vi "LeCroy Test Driver V2.vi"() -> ()   [LabVIEW 2013]
doc: "This example shows how to configure the oscilloscope to perform an edge-triggered waveform acquisition."
uses:
  Sub VI's/Settings_TypeDef.ctl
  <instrlib>/LeCroy Wave Series/LeCroy Wave Series.lvlib
panel:
  in  "Settings":T1={"LeCroy IP"="169.254.20.90", "Ch1"={"On/Off"=FALSE, "Bandwidth (Dropdown)"=0, "Vertical Range (V)"=0.2, "Vertical Offset (V)"=0.0}, "Ch2"={"On/Off"=TRUE, "Bandwidth (Dropdown)"=0, "Vertical Range (V)"=1.2, "Vertical Offset (V)"=0.0}, "Ch3"={"On/Off"=TRUE, "Bandwidth (Dropdown)"=0, "Vertical Range (V)"=0.2, "Vertical Offset (V)"=0.0}, "Ch4"={"On/Off"=FALSE, "Bandwidth (Dropdown)"=0, "Vertical Range (V)"=0.2, "Vertical Offset (V)"=0.0}, "T axis"={"Time base (s/div)"=0.0002, "Time offset (s)"=0.0, "Max Sample Points"=5000}, "Trig"={"Trigger mode"=2, "Trigger Slope"=0, "Trigger Source"=1, "Trigger Level (V)"=0.04}, "Timeout (ms)"=10000.0} {"Trig"."Trigger mode" items=["Auto", "Normal", "Single", "Single, auto trigger"]; "Trig"."Trigger Slope" items=["Rising", "Falling"]; "Trig"."Trigger Source" items=["Channel 1", "Channel 2", "Channel 3", "Channel 4", "External", "Power Line"]; "Trig"."Trigger Level (V)" format="%#_6p"; "T axis"."Max Sample Points" format="%.0p" items=["50"=50, "100"=100, "250"=250, "500"=500, "1000"=1000, "2500"=2500, "5K"=5000, "10K"=10000, "25K"=25000, "50K"=50000, "100K"=100000, "250K"=250000, "500K"=500000, "1M"=1000000, "2M"=2000000, "2.5M"=2500000, "5M"=5000000, "10M"=10000000, "25M"=25000000, "50M"=50000000, "100M"=100000000]; "T axis"."Time base (s/div)" format="%#_6p"; "Ch4"."Bandwidth (Dropdown)" items=["Full", "20MHZ", "25MHZ", "200MHZ", "250MHZ", "1GHZ", "3GHZ", "4GHZ"]; "Ch3"."Bandwidth (Dropdown)" items=["Full", "20MHZ", "25MHZ", "200MHZ", "250MHZ", "1GHZ", "3GHZ", "4GHZ"]; "Ch2"."Bandwidth (Dropdown)" items=["Full", "20MHZ", "25MHZ", "200MHZ", "250MHZ", "1GHZ", "3GHZ", "4GHZ"]; "Ch1"."Bandwidth (Dropdown)" items=["Full", "20MHZ", "25MHZ", "200MHZ", "250MHZ", "1GHZ", "3GHZ", "4GHZ"]}
  out "Configure time (ms)":u32
  out "Initilize time (ms)":u32
  out "Aquire waveform time (ms)":u32
  out "Waveform Data":waveform(dbl)[](graph)
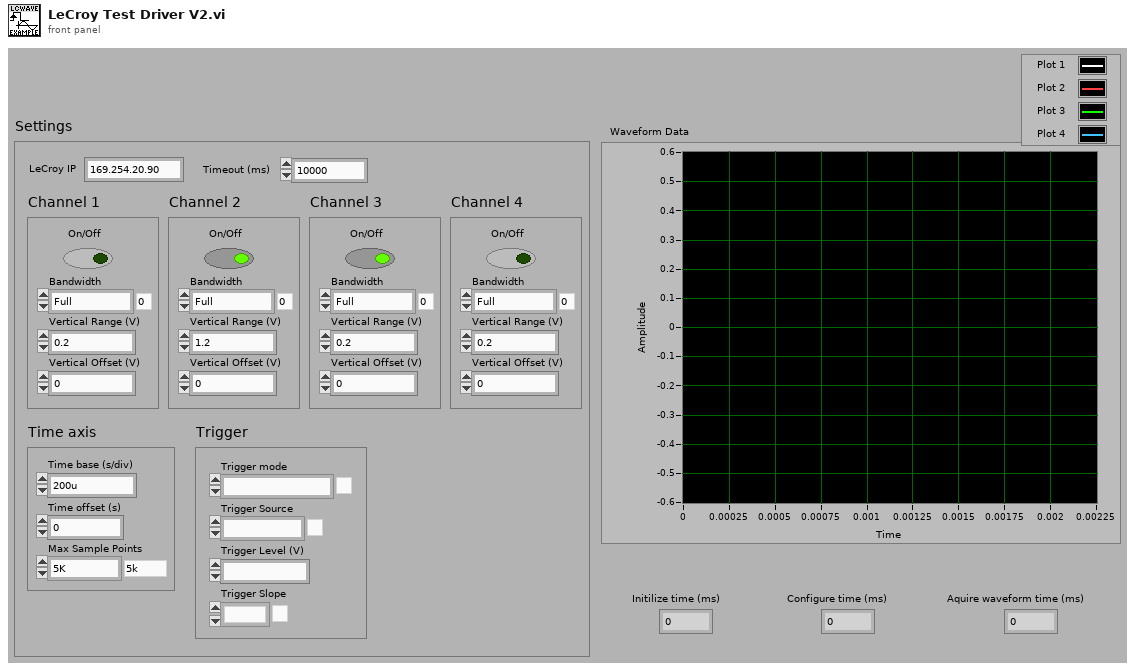
[diagram p1: front panel]
types:
  T1 = typedef "Settings_TypeDef.ctl" = cluster{"LeCroy IP":string, "Ch1":cluster{"On/Off":bool, "Bandwidth (Dropdown)":u16, "Vertical Range (V)":dbl, "Vertical Offset (V)":dbl}, "Ch2":cluster{"On/Off":bool, "Bandwidth (Dropdown)":u16, "Vertical Range (V)":dbl, "Vertical Offset (V)":dbl}, "Ch3":cluster{"On/Off":bool, "Bandwidth (Dropdown)":u16, "Vertical Range (V)":dbl, "Vertical Offset (V)":dbl}, "Ch4":cluster{"On/Off":bool, "Bandwidth (Dropdown)":u16, "Vertical Range (V)":dbl, "Vertical Offset (V)":dbl}, "T axis":cluster{"Time base (s/div)":dbl, "Time offset (s)":dbl, "Max Sample Points":i32}, "Trig":cluster{"Trigger mode":u16, "Trigger Slope":u16, "Trigger Source":u16, "Trigger Level (V)":dbl}, "Timeout (ms)":dbl}
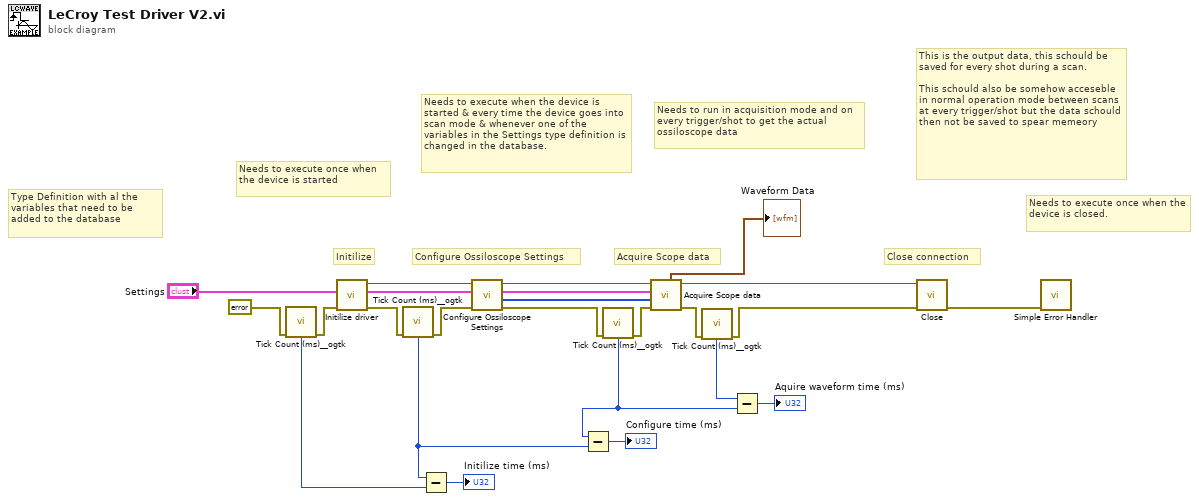
[diagram p0: block diagram]
diagram:
  # "Needs to execute once when the device is closed."
  # "This is the output data, this schould be saved for every shot during a scan.\n\nThis schould also be somehow acceseble in normal operation mode between scans at every trigger/shot but the data schould then not be saved to spear memeory"
  # "Needs to run in acquisition mode and on every trigger/shot to get the actual ossiloscope data"
  # "Needs to execute when the device is started & every time the device goes into scan mode & whenever one of the variables in the Settings type definition is changed in the database."
  # "Needs to execute once when the device is started"
  # "Type Definition with al the variables that need to be added to the database"
  # "Close connection"
  # "Acquire Scope data"
  # "Configure Ossiloscope Settings"
  # "Initilize"
  n1 = call <userlib>:"Tick Count (ms)__ogtk.vi"("error in (no error)"=errorcluster {"status"=FALSE, "code"=0, "source"=""} ("error in")) -> ("error out"=w8:errorcluster, "millisecond timer value"=w5:u32)  [unwired: 9 in]
  n2 = call "Initilize driver.vi"("error in"=w8, "input settings"="Settings") -> ("error out"=w10:errorcluster, "output settings"=w19:T1, "VISA resource name out"=w20:refnum<visa-resource-name>)  [unwired: 7 in]
  n3 = call <userlib>:"Tick Count (ms)__ogtk.vi"("error in (no error)"=w10) -> ("error out"=w11:errorcluster, "millisecond timer value"=w4:u32)  [unwired: 9 in]
  n4 = Subtract(x=w4, y=w5) -> (x-y=→"Initilize time (ms)":u32)
  n5 = call "Configure Ossiloscope Settings.vi"("error in"=w11, "input settings"=w19, "VISA resource name in"=w20) -> ("error out"=w18:errorcluster, "Channels to read out"=w13:i32[], "output settings"=w2:T1, "VISA resource name out"=w15:refnum<visa-resource-name>)  [unwired: 5 in]
  n6 = call <userlib>:"Tick Count (ms)__ogtk.vi"("error in (no error)"=w18) -> ("error out"=w16:errorcluster, "millisecond timer value"=w3:u32)  [unwired: 9 in]
  n7 = Subtract(x=w3, y=w4) -> (x-y=→"Configure time (ms)":u32)
  n8 = call "Acquire Scope data.vi"("error in"=w16, "Channels to read in"=w13, "input settings"=w2, "VISA resource name in"=w15) -> ("error out"=w17:errorcluster, "VISA resource name out"=w14:refnum<visa-resource-name>, "Waveform Data out"=→"Waveform Data":waveform(dbl)[])  [unwired: 4 in, 1 out]
  n9 = call <userlib>:"Tick Count (ms)__ogtk.vi"("error in (no error)"=w17) -> ("error out"=w23:errorcluster, "millisecond timer value"=w22:u32)  [unwired: 9 in]
  n10 = Subtract(x=w22, y=w3) -> (x-y=→"Aquire waveform time (ms)":u32)
  n11 = call <instrlib>:"Close.vi"("error in (no error)"=w23, "VISA resource name"=w14) -> ("error out"=w24:errorcluster)  [unwired: 9 in]
  n12 = call <vilib>:"Simple Error Handler.vi"("error in (no error)"=w24) -> ()  [unwired: 4 in, 5 out]
